vi "Intake IR.vi"(11 "Speed":dbl) -> (3 "Speeeeeeed":dbl)   [LabVIEW 2015]
uses:
  Common Code/Intake Commands Cluster.ctl
  Common Code/Intake Commands.ctl
  Common Code/Intake Mode.ctl
panel:
  in  "Intake Commands Cluster":T1={"Intake Commands"=enum."Load", "Intake Mode"=enum."Auto", "Override IR"=FALSE}
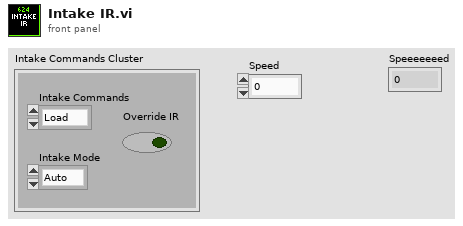
[diagram p1: front panel]
types:
  T1 = typedef "Intake Commands Cluster.ctl" = cluster{"Intake Commands":T2, "Intake Mode":T3, "Override IR":bool}
  T2 = typedef "Intake Commands.ctl" = enum16{"Unload", "Load", "Pull up", "Drop low", "Idle", "Lift Half"}
  T3 = typedef "Intake Mode.ctl" = enum16{"Safe", "Auto", "Manual"}
  T4 = typedef "WPI_DigitalInputDevRef.ctl" = cluster{"DevStatus":errorcluster, "DIO Channel":T5}
  T5 = typedef "FPGA_DIOChannel.ctl" = enum8{"DIO 0", "DIO 1", "DIO 2", "DIO 3", "DIO 4", "DIO 5", "DIO 6", "DIO 7", "DIO 8", "DIO 9", "DIO MXP 0", "DIO MXP 1", "DIO MXP 2", "DIO MXP 3", "DIO MXP 4", "DIO MXP 5", "DIO MXP 6", "DIO MXP 7", "DIO MXP 8", "DIO MXP 9", "DIO MXP 10", "DIO MXP 11", "DIO MXP 12", "DIO MXP 13", "DIO MXP 14", "DIO MXP 15", "Invalid"}
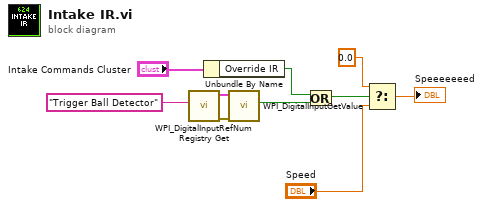
[diagram p0: block diagram]
diagram:
  n1 = call <vilib>:"WPI_DigitalInputRefNum Registry Get.vi"("refnum name"="Trigger Ball Detector") -> ("error out"=w9:errorcluster, "DigitalInputDevRef"=w8:T4)  [unwired: 9 in]
  n2 = Unbundle By Name("Intake Commands Cluster") -> ("Override IR"=w4:bool)
  n3 = call <vilib>:"WPI_DigitalInputGetValue.vi"("error in (no error)"=w9, "DigitalInputDevRef"=w8) -> ("Value"=w5:bool)  [unwired: 7 in, 2 out]
  n4 = Or(x=w4, y=w5) -> (x .or. y?=w6:bool)
  n5 = Select(t=0.0, s=w6, f="Speed") -> (s? t:f=→"Speeeeeeed":dbl)
